vi "Execute.vi"(8 "Error In":errorcluster, 11 "Error Handling In":refnum<class "Error Handling.lvclass">) -> (0 "Error Out":errorcluster, 3 "Error Handling Out":refnum<class "Error Handling.lvclass">)   [LabVIEW 2019, in "Error Handling.lvclass"]
uses:
  Error Handling.lvclass
  C:/Users/goo13/Documents/GIT Local/myDashBoard/Source/RT/Process/Process.lvclass
  Process/Process.lvclass
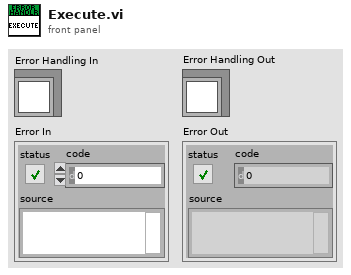
[diagram p1: front panel]
types:
  T1 = typedef "Process.lvclass/Process Message.ctl" = cluster{"Command":string, "Data":variant}
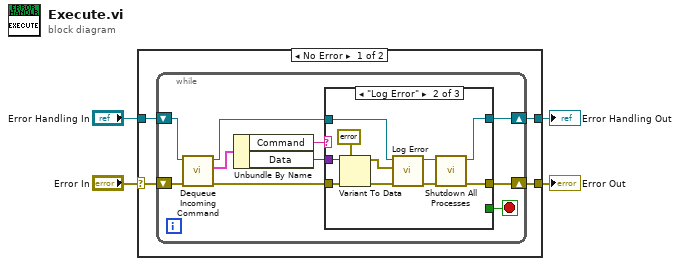
[diagram p0: block diagram]
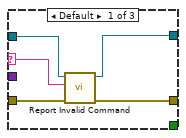
[diagram p2: hidden frame]
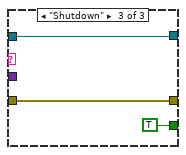
[diagram p3: hidden frame]
diagram:
  n1 = case shown="No Error" "Error In" {
    selector: "Error In" -> [w7 w38]
    tunnel: [w8 w38] -> w3
    tunnel: "Error Handling In" -> [w6 w37]
    tunnel: [w5 w37] -> w1
    frame No Error {
      n2 = while {
        shift-right: [w11] -> w8
        shift-left: w7 -> [w18]
        shift-right: [w9] -> w5
        shift-left: w6 -> [w17]
        stop <- w10 stop-if-true
        n3 = call "Dequeue Incoming Command.vi"("Error In"=w18, "Process In"=w17) -> ("Error Out"=w13:errorcluster, "Process Message"=w16:T1, "Process Out"=w14:refnum<class "Error Handling.lvclass">)  [unwired: 7 in]
        n4 = Unbundle By Name(w16) -> ("Command"=w15:string, "Data"=w12:variant)
        n5 = case shown="\"Log Error\"" w15 {
          selector: w15 -> [w21 _ _]
          tunnel: w14 -> [w23 w33 w34]
          tunnel: w13 -> [w22 w31 w36]
          tunnel: w12 -> [_ w32 _]
          tunnel: [w19 w24 w36] -> w11
          tunnel: [_ _ TRUE] -> w10
          tunnel: [w20 w25 w34] -> w9
          frame Default {
            n6 = call "Report Invalid Command.vi"("Error In"=w22, "Command"=w21, "Process In"=w23) -> ("Error Out"=w19:errorcluster, "Process Out"=w20:refnum<class "Error Handling.lvclass">)  [unwired: 7 in]
          }
          frame "Log Error" {
            n7 = Variant To Data(error in=w31, type=errorcluster {"status"=FALSE, "code"=0, "source"=""} ("Error To Log"), Variant=w32) -> (data=w30:errorcluster, error out=w29:errorcluster)
            n8 = call "Log Error.vi"("Error In"=w29, "Error To Log"=w30, "Error Handling In"=w33) -> ("Error Out"=w26:errorcluster, "Error Handling Out"=w27:refnum<class "Error Handling.lvclass">)  [unwired: 7 in]
            n9 = call "Shutdown All Processes.vi"("Error In"=w26, "Error Handling In"=w27) -> ("Error Out"=w24:errorcluster, "Error Handling Out"=w25:refnum<class "Error Handling.lvclass">)  [unwired: 8 in]
          }
          frame "Shutdown" {
          }
        }
      }
    }
    frame Error {
    }
  }
  "Error Out" <- w3
  "Error Handling Out" <- w1
